vi "ResetAlarm.vi"(4 "LineName":string, 6 "ConnectionDSN":string, 8 "ArrayAlarmIN":bool[](array[boolean]), 9 "PLC Connection Array":T1(array[cluster]) {"PLC Type" items=["Keyence", "Allen Bradley", "Mitsubishi", "Panasonic", "Siemens"]}, 10 "OnlineStations":T3(array[cluster]), 11 "Counters Monitor Array IN":T2(array[cluster])) -> (0 "ArrayAlarmOUT":bool[](array[boolean]), 1 "Counters Monitor Array OUT":T2(array[cluster]))   [LabVIEW 2017]
panel:
  in  "Comments":string
  in  "EWOFolio":string
  in  "ToolCribFolio":string
  out "ArrayIncidenceID":string[](array[string])
  out "IncidenceID":dbl
  in  "Reset":bool
  in  "Components List":u16(ring) items=["MA520 replace the component: componente de miguel - 101111", "MA475 replace the component: spinning belt - 104567", "MA500-3 replace the component: component1 - 131415", "MA530 replace the component: componente2 - 181717", "MA530 replace the component: component3 - 181716", "MA520 replace the component: helicoil - 105855", "MA520 replace the component: newpart - 101415", "MA500-3 replace the component: component2 - 141516", "MA500-2 replace the component: component1 - 151617", "MA500-2 replace the component: component2 - 171819", "MA500-1 replace the component: component1 - 141516", "MA490-2 replace the component: component1 - 121314", "MA490-1 replace the component: component1 - 161718", "MA470 replace the component: electrodes - 121314", "MA455 replace the component: component1 - 191817"]
  # "Please, select the component you'd like to reset."
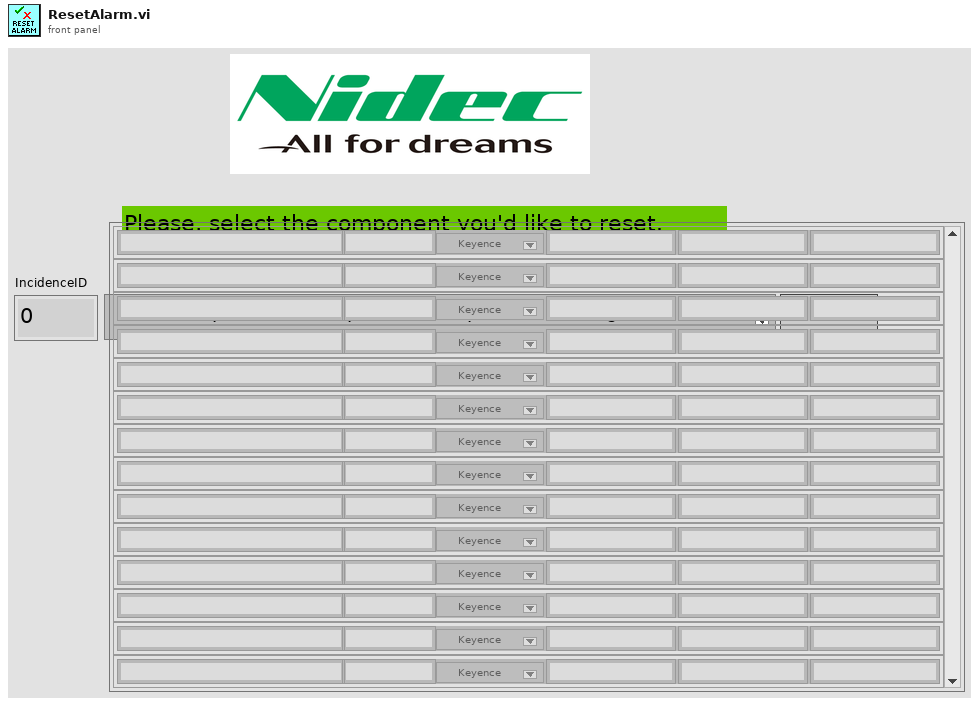
[diagram p1: front panel]
types:
  T1 = cluster{"MachineName":string, "PLC Address":string, "PLC Type":u16, "MemoryNumber1":string, "MemoryNumber2":string, "MemoryNumber3":string}[]
  T2 = cluster{"MachineName":string, "ComponentName":string, "StoppageAlarmCounter":i32, "CurrentCount":i32, "StatusColorBox":u32, "ToolCribPartNumber":string}[]
  T3 = cluster{"Connection":bool, "MachineName":string}[]
  T4 = cluster{"MachineName":string, "ComponentName":string, "StoppageAlarmCounter":i32, "CurrentCount":i32, "StatusColorBox":u32, "ToolCribPartNumber":string}
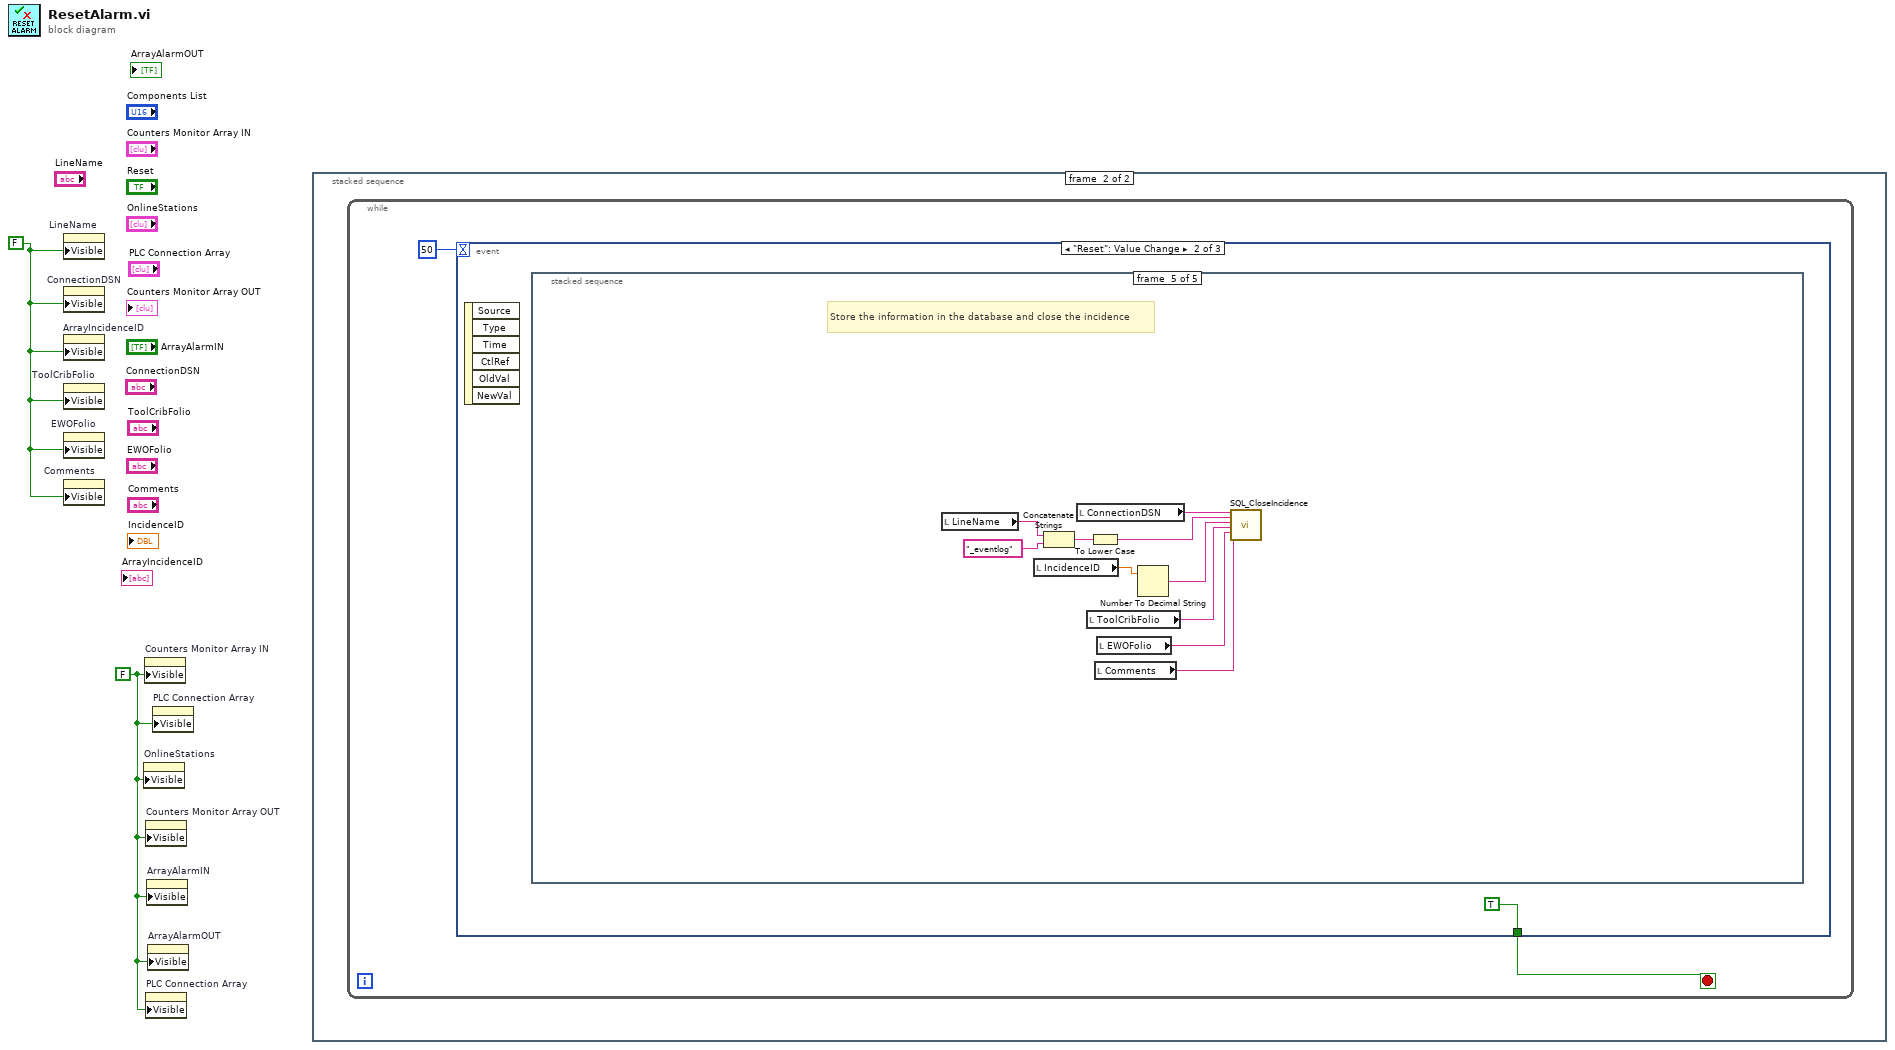
[diagram p0: block diagram]
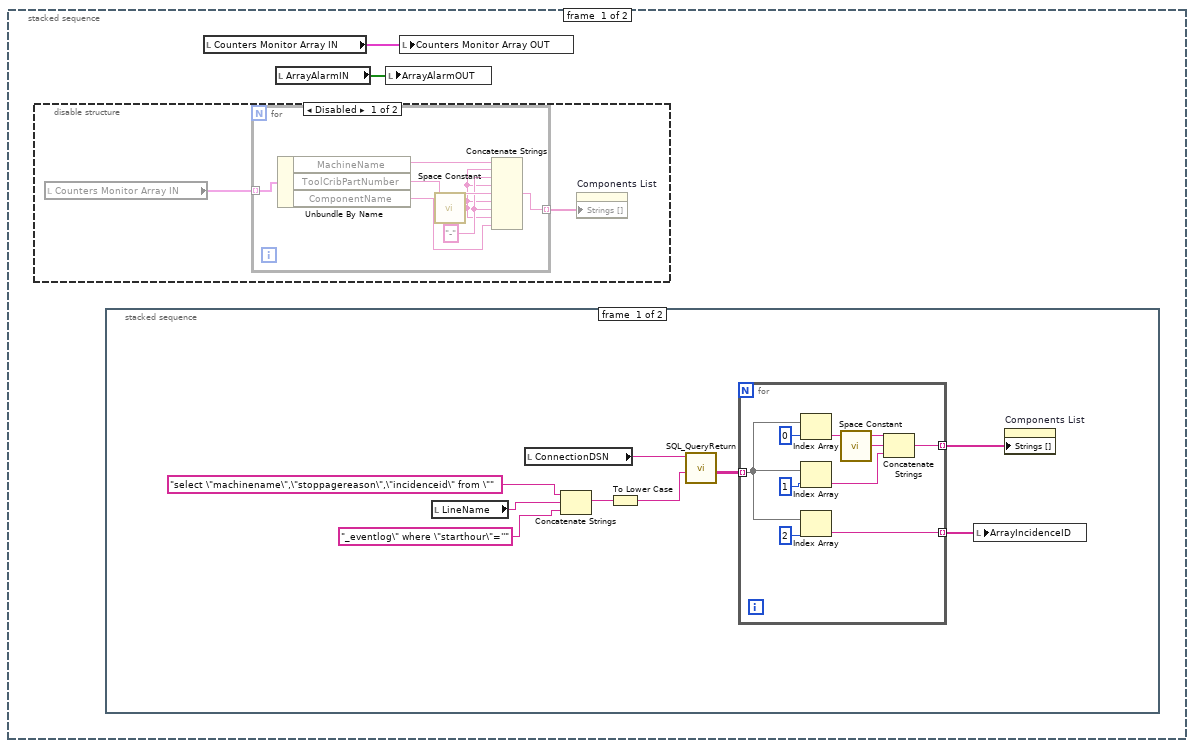
[diagram p2: hidden frame]
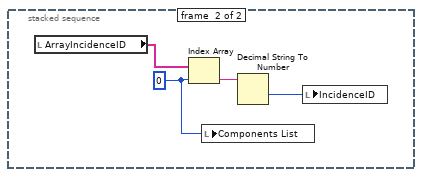
[diagram p3: hidden frame]
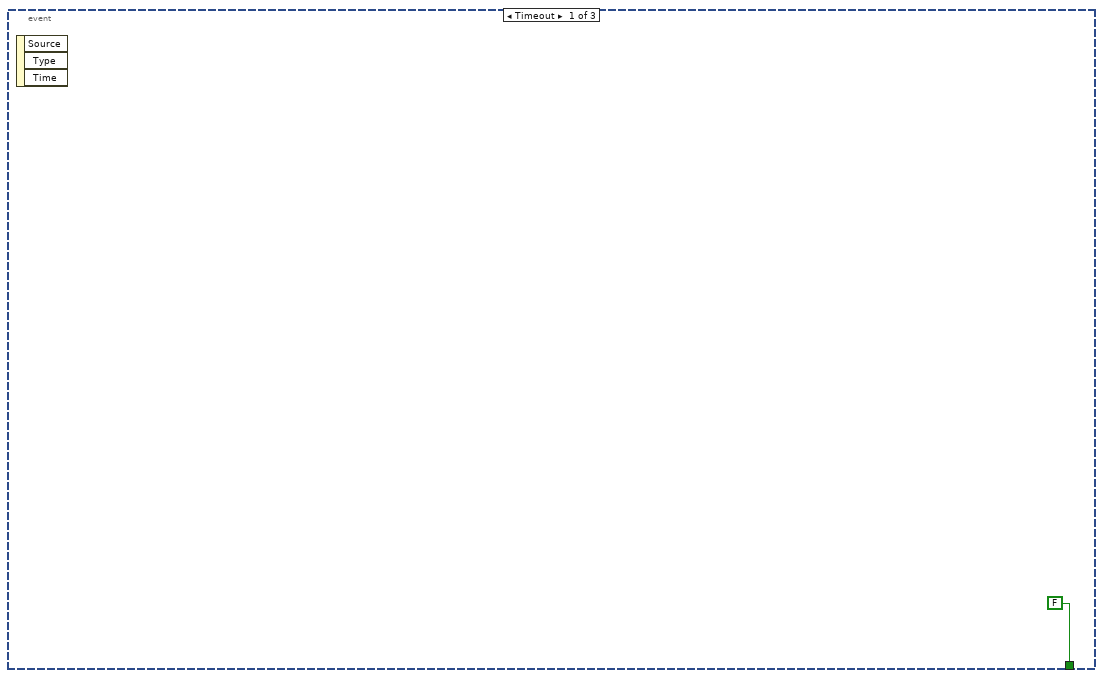
[diagram p5: hidden frame]
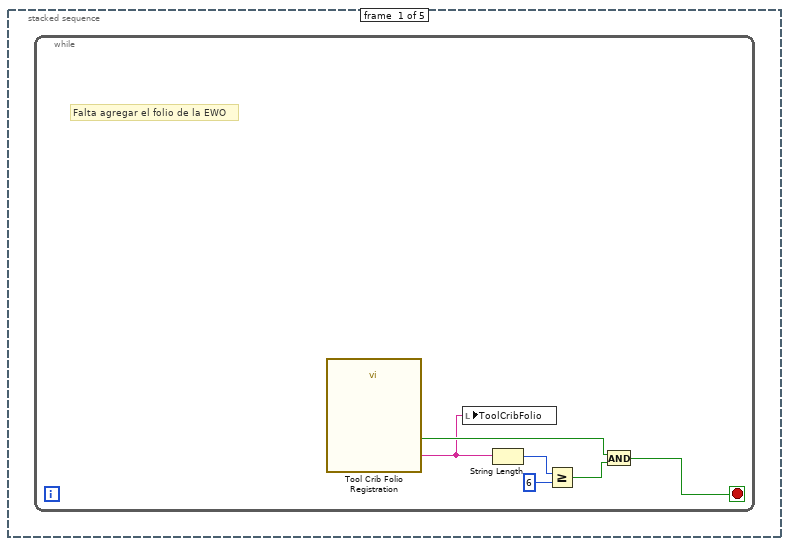
[diagram p6: hidden frame]
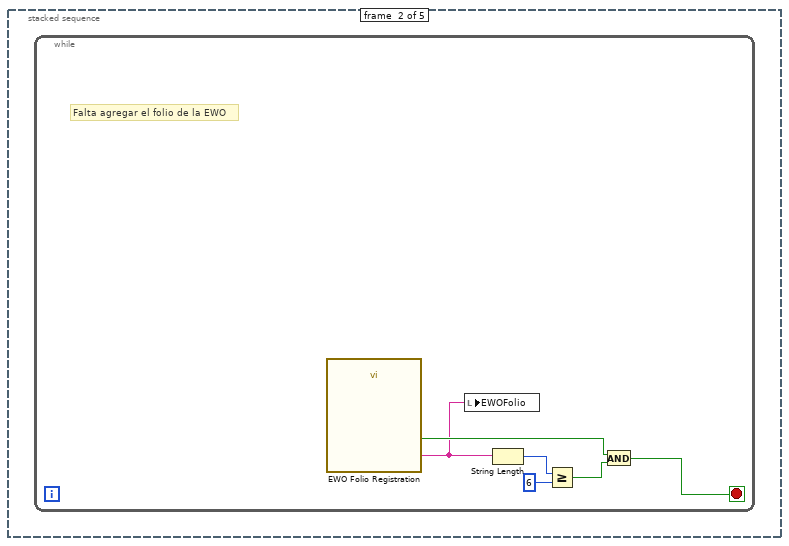
[diagram p7: hidden frame]
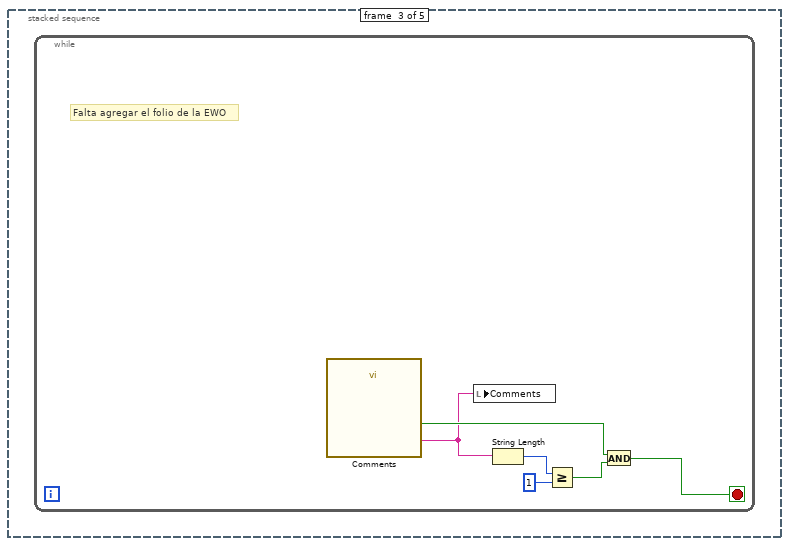
[diagram p8: hidden frame]
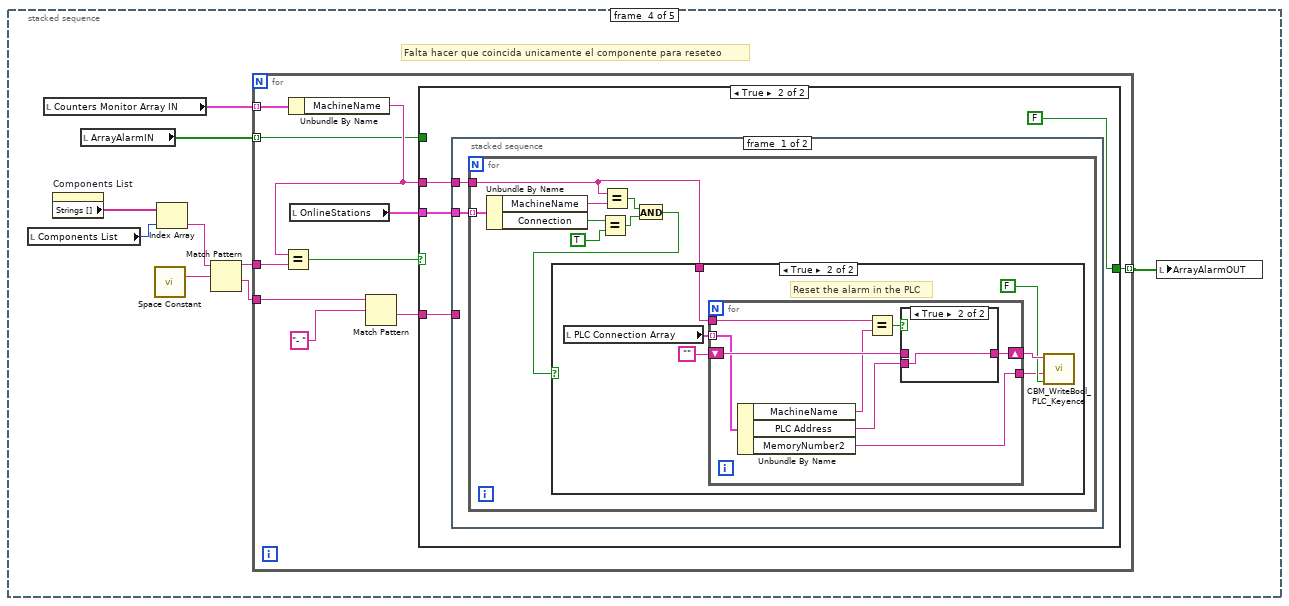
[diagram p9: hidden frame]
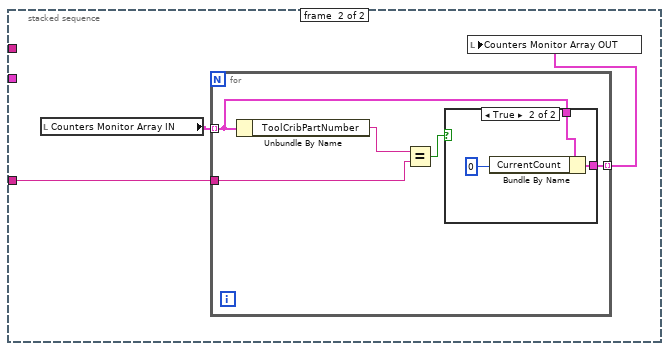
[diagram p13: hidden frame]
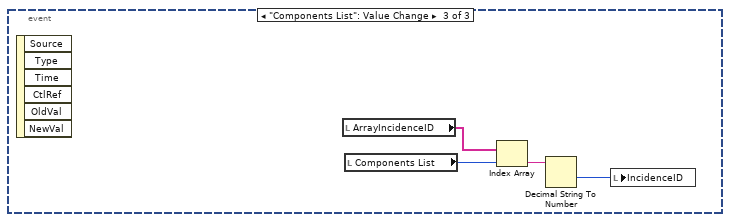
[diagram p15: hidden frame]
diagram:
  w2 = FALSE
  w1 = FALSE
  n1 = property on="LineName" class="Str"("Visible"=w2) -> ()  [unwired: 2 in, 2 out]
  n2 = property on="ConnectionDSN" class="Str"("Visible"=w2) -> ()  [unwired: 2 in, 2 out]
  n3 = property on="ArrayIncidenceID" class="Arr (strict)"("Visible"=w2) -> ()  [unwired: 2 in, 2 out]
  n4 = property on="ToolCribFolio" class="Str"("Visible"=w2) -> ()  [unwired: 2 in, 2 out]
  n5 = property on="EWOFolio" class="Str"("Visible"=w2) -> ()  [unwired: 2 in, 2 out]
  n6 = property on="Comments" class="Str"("Visible"=w2) -> ()  [unwired: 2 in, 2 out]
  n7 = property on="OnlineStations" class="Arr (strict)"("Visible"=w1) -> ()  [unwired: 2 in, 2 out]
  n8 = property on="Counters Monitor Array IN" class="Arr (strict)"("Visible"=w1) -> ()  [unwired: 2 in, 2 out]
  n9 = property on="Counters Monitor Array OUT" class="Arr (strict)"("Visible"=w1) -> ()  [unwired: 2 in, 2 out]
  n10 = property on="PLC Connection Array" class="Arr (strict)"("Visible"=w1) -> ()  [unwired: 2 in, 2 out]
  n11 = property on="ArrayAlarmIN" class="Arr (strict)"("Visible"=w1) -> ()  [unwired: 2 in, 2 out]
  n12 = property on="ArrayAlarmOUT" class="Arr (strict)"("Visible"=w1) -> ()  [unwired: 2 in, 2 out]
  n13 = property on="PLC Connection Array" class="Arr (strict)"("Visible"=w1) -> ()  [unwired: 2 in, 2 out]
  n14 = stacked-sequence {
    frame #0 {
      n15 = disable-structure shown="Disabled" {
        frame Disabled {
          n16 = local read "Counters Monitor Array IN"() -> (w28:T2)
          n17 = for {
            tunnel: [w33] -> w27 mode=indexing
            tunnel: w28 -> [w32] mode=indexing
            w31 = "-"
            n18 = Unbundle By Name(w32) -> ("MachineName"=w29:string, "ToolCribPartNumber"=w35:string, "ComponentName"=w34:string)
            n19 = call <vilib>:"Space Constant.vi"() -> ("String"=w30:string)
            n20 = Concatenate Strings(w29, w30, w31, w30, w35, w30, w31, w30, w34) -> (w33:string)
          }
          n21 = property on="Components List" class="Ring (strict)"("Strings []"=w27) -> ()  [unwired: 2 in, 2 out]
        }
        frame Enabled {
        }
      }
      n22 = stacked-sequence {
        frame #0 {
          n23 = local read "LineName"() -> (w11:string)
          n24 = local read "ConnectionDSN"() -> (w13:string)
          n25 = Concatenate Strings("select \"machinename\",\"stoppagereason\",\"incidenceid\" from \"" ("SQL query"), w11, "_eventlog\" where \"starthour\"=''" ("SQL query")) -> (w9:string)
          n26 = To Lower Case(string=w9) -> (all lower case string=w8:string)
          n27 = call "SQL_QueryReturn.vi"("SQL query"=w8, "ConnectionDSN"=w13) -> ("data"=w7:string[][])  [unwired: 9 in]
          n28 = for {
            tunnel: w7 -> [w15] mode=indexing
            tunnel: [w17] -> w6 mode=indexing
            tunnel: [w14] -> w5 mode=indexing
            n29 = Index Array(array=w15, index=0) -> (element=w20:string)
            n30 = Index Array(array=w15, index=1) -> (element=w19:string)
            n31 = Index Array(array=w15, index=2) -> (element=w14:string)
            n32 = call <vilib>:"Space Constant.vi"() -> ("String"=w18:string)
            n33 = Concatenate Strings(w20, w18, w19) -> (w17:string)
          }
          n34 = local write "ArrayIncidenceID"(w5) -> ()
          n35 = property on="Components List" class="Ring (strict)"("Strings []"=w6) -> ()  [unwired: 2 in, 2 out]
        }
        frame #1 {
          w23 = 0 ("index")
          n36 = local read "ArrayIncidenceID"() -> (w24:string[])
          n37 = Index Array(array=w24, index=w23) -> (element=w25:string)
          n38 = local write "Components List"(w23) -> ()
          n39 = Decimal String To Number(string=w25) -> (number=w26:i32)  [unwired: 2 in, 1 out]
          n40 = local write "IncidenceID"(w26) -> ()
        }
      }
      n41 = local read "Counters Monitor Array IN"() -> (w4:T2)
      n42 = local read "ArrayAlarmIN"() -> (w3:bool[])
      n43 = local write "ArrayAlarmOUT"(w3) -> ()
      n44 = local write "Counters Monitor Array OUT"(w4) -> ()
    }
    frame #1 {
      n45 = while {
        stop <- w36 stop-if-true
        n46 = event shown="[1] \"Reset\": Value Change" {
          selector: _ -> [_ _ _]
          dyn-events: _ -> [_ _ _]
          timeout: 50 -> [_ _ _]
          tunnel: [FALSE TRUE _] -> w36
          event Timeout {
            n47 = event-data() -> ()  [unwired: 1 in, 3 out]
          }
          event "Reset": Value Change {
            n48 = event-data() -> ()  [unwired: 1 in, 6 out]
            n49 = stacked-sequence {
              frame #0 {
                n50 = while {
                  stop <- w41 stop-if-true
                  # "Falta agregar el folio de la EWO"
                  n51 = call "Tool Crib Folio Registration"() -> ("ToolCrib Folio"=w40:string, "OK"=w42:bool)  [unwired: 17 in, 1 out]
                  n52 = local write "ToolCribFolio"(w40) -> ()
                  n53 = String Length(string=w40) -> (length=w45:i32)
                  n54 = Greater Or Equal?(x=w45, y=6) -> (x >= y?=w43:bool)
                  n55 = And(x=w42, y=w43) -> (x .and. y?=w41:bool)
                }
              }
              frame #1 {
                n56 = while {
                  stop <- w47 stop-if-true
                  # "Falta agregar el folio de la EWO"
                  n57 = call "EWO Folio Registration"() -> ("EWO Folio"=w46:string, "OK"=w48:bool)  [unwired: 17 in, 1 out]
                  n58 = local write "EWOFolio"(w46) -> ()
                  n59 = String Length(string=w46) -> (length=w51:i32)
                  n60 = Greater Or Equal?(x=w51, y=6) -> (x >= y?=w49:bool)
                  n61 = And(x=w48, y=w49) -> (x .and. y?=w47:bool)
                }
              }
              frame #2 {
                n62 = while {
                  stop <- w53 stop-if-true
                  # "Falta agregar el folio de la EWO"
                  n63 = call "Comments"() -> ("Comments"=w52:string, "OK"=w54:bool)  [unwired: 17 in, 1 out]
                  n64 = local write "Comments"(w52) -> ()
                  n65 = String Length(string=w52) -> (length=w57:i32)
                  n66 = Greater Or Equal?(x=w57, y=1) -> (x >= y?=w55:bool)
                  n67 = And(x=w54, y=w55) -> (x .and. y?=w53:bool)
                }
              }
              frame #3 {
                # "Falta hacer que coincida unicamente el componente para reseteo"
                n68 = local read "Components List"() -> (w64:u16)
                n69 = local read "Counters Monitor Array IN"() -> (w66:T2)
                n70 = property on="Components List" class="Ring (strict)"() -> ("Strings []"=w65:string[])  [unwired: 2 in, 2 out]
                n71 = local read "ArrayAlarmIN"() -> (w60:bool[])
                n72 = call <vilib>:"Space Constant.vi"() -> ("String"=w62:string)
                n73 = Index Array(array=w65, index=w64) -> (element=w63:string)
                n74 = Match Pattern(string=w63, regular expression=w62) -> (before substring=w61:string, after substring=w58:string)  [unwired: 1 in, 2 out]
                n75 = for {
                  tunnel: w66 -> [w70] mode=indexing
                  tunnel: w61 -> [w75]
                  tunnel: w60 -> [w72] mode=indexing
                  tunnel: [w71] -> w59 mode=indexing
                  tunnel: w58 -> [w69]
                  n76 = Unbundle By Name(w70) -> ("MachineName"=w74:string)
                  n77 = Equal?(x=w74, y=w75) -> (x = y?=w73:bool)
                  n78 = local read "OnlineStations"() -> (w76:T3)
                  n79 = Match Pattern(string=w69, regular expression="- ") -> (after substring=w67:string)  [unwired: 1 in, 3 out]
                  n80 = case shown="True" w73 {
                    tunnel: w76 -> [_ w81]
                    tunnel: w74 -> [_ w80]
                    tunnel: w72 -> [w77 _]
                    tunnel: [w77 FALSE] -> w71
                    tunnel: w67 -> [_ w79]
                    frame False {
                    }
                    frame True {
                      n81 = stacked-sequence {
                        tunnel: w81 -> [w83 _]
                        tunnel: w80 -> [w82 _]
                        tunnel: w79 -> [_ w110]
                        frame #0 {
                          n82 = for {
                            tunnel: w82 -> [w89]
                            tunnel: w83 -> [w91] mode=indexing
                            n83 = Unbundle By Name(w91) -> ("MachineName"=w90:string, "Connection"=w88:bool)
                            n84 = Equal?(x=w88, y=TRUE) -> (x = y?=w86:bool)
                            n85 = Equal?(x=w89, y=w90) -> (x = y?=w85:bool)
                            n86 = And(x=w85, y=w86) -> (x .and. y?=w84:bool)
                            n87 = case shown="True" w84 {
                              tunnel: w89 -> [_ w93]
                              frame False {
                              }
                              frame True {
                                # "Reset the alarm in the PLC"
                                n88 = local read "PLC Connection Array"() -> (w96:T1)
                                n89 = for {
                                tunnel: w96 -> [w100] mode=indexing
                                tunnel: w93 -> [w105]
                                shift-right: [w102] -> w97
                                shift-left: "" -> [w101]
                                tunnel: [w99] -> w92
                                n90 = Unbundle By Name(w100) -> ("MachineName"=w98:string, "PLC Address"=w103:string, "MemoryNumber2"=w99:string)
                                n91 = Equal?(x=w105, y=w98) -> (x = y?=w104:bool)
                                n92 = case shown="True" w104 {
                                tunnel: w103 -> [_ w107]
                                tunnel: [w106 w107] -> w102
                                tunnel: w101 -> [w106 _]
                                frame False {
                                }
                                frame True {
                                }
                                }
                                }
                                n93 = call "CBM_WriteBool_PLC_Keyence.vi"("Set?"=FALSE, "MemoryNumber"=w92, "PLC_IP"=w97) -> ()  [unwired: 8 in, 1 out]
                              }
                            }
                          }
                        }
                        frame #1 {
                          n94 = local read "Counters Monitor Array IN"() -> (w109:T2)
                          n95 = for {
                            tunnel: w109 -> [w113] mode=indexing
                            tunnel: w110 -> [w114]
                            tunnel: [w111] -> w108 mode=indexing
                            n96 = Unbundle By Name(w113) -> ("ToolCribPartNumber"=w115:string)
                            n97 = Equal?(x=w115, y=w114) -> (x = y?=w112:bool)
                            n98 = case shown="True" w112 {
                              tunnel: w113 -> [w116 w119]
                              tunnel: [w116 w117] -> w111
                              frame False {
                              }
                              frame True {
                                n99 = Bundle By Name(cluster=w119, "CurrentCount"=0) -> (w117:T4)
                              }
                            }
                          }
                          n100 = local write "Counters Monitor Array OUT"(w108) -> ()
                        }
                      }
                    }
                  }
                }
                n101 = local write "ArrayAlarmOUT"(w59) -> ()
              }
              frame #4 {
                # "Store the information in the database and close the incidence"
                n102 = local read "LineName"() -> (w128:string)
                n103 = local read "IncidenceID"() -> (w124:dbl)
                n104 = Concatenate Strings(w128, "_eventlog" ("SQL query")) -> (w126:string)
                n105 = local read "ConnectionDSN"() -> (w129:string)
                n106 = local read "ToolCribFolio"() -> (w122:string)
                n107 = To Lower Case(string=w126) -> (all lower case string=w125:string)
                n108 = local read "Comments"() -> (w120:string)
                n109 = local read "EWOFolio"() -> (w121:string)
                n110 = Number To Decimal String(number=w124) -> (decimal integer string=w123:string)  [unwired: 1 in]
                n111 = call "SQL_CloseIncidence.vi"("ConnectionDSN"=w129, "TableName"=w125, "IncidenceID"=w123, "ToolCribFolio"=w122, "EWOFolio"=w121, "Comments"=w120) -> ()  [unwired: 14 in]
              }
            }
          }
          event "Components List": Value Change {
            n112 = event-data() -> ()  [unwired: 1 in, 6 out]
            n113 = local read "ArrayIncidenceID"() -> (w132:string[])
            n114 = local read "Components List"() -> (w133:u16)
            n115 = Index Array(array=w132, index=w133) -> (element=w131:string)
            n116 = Decimal String To Number(string=w131) -> (number=w130:i32)  [unwired: 2 in, 1 out]
            n117 = local write "IncidenceID"(w130) -> ()
          }
        }
      }
    }
  }
